vi "UPGRADE_Surge IFSM.vi"() -> ()   [LabVIEW 2019]
uses:
  <vilib>/Utility/NIReport.llb/Report Type.ctl
  <vilib>/Utility/NIReport.llb/NI_report.lvclass
  <vilib>/Utility/NIReport.llb/NI_ReportGenerationCore.lvlib
  <vilib>/Utility/NIReport.llb/Excel/NI_Excel.lvclass
panel:
  in  "Lot ID":string
  in  "Direction":string(combo)
  in  "Frequency (Hz)":i32
  in  "Temperature (+)":i32
  in  "Device ID":string
  in  "Technician":string
  in  "Request Number":i32
  out "STEP 8":bool
  out "STEP 7":bool
  out "STEP 6":bool
  out "STEP 5":bool
  in  "START Button":bool
  out "STEP 4":bool
  out "STEP 3":bool
  out "STEP 2":bool
  out "STEP 1":bool
  in  "FILE PATH":path
  # "DATA SUMMARY FOR SURGE IFSM"
  # "OPEN EXCEL FILE"
  # "RUN MACRO INTO EXCEL FILE"
  # "Create New Sheet named (Request Number_Surge_IFSM)"
  # "Create Table named (\"Last  Good Pass\")"
  # "Create New Sheet and Table named (\"Summary Table\")"
  # "Move All Tabs into a new Excel Workbook"
  # "SAVE EXCEL FILE"
  # "FINISH"
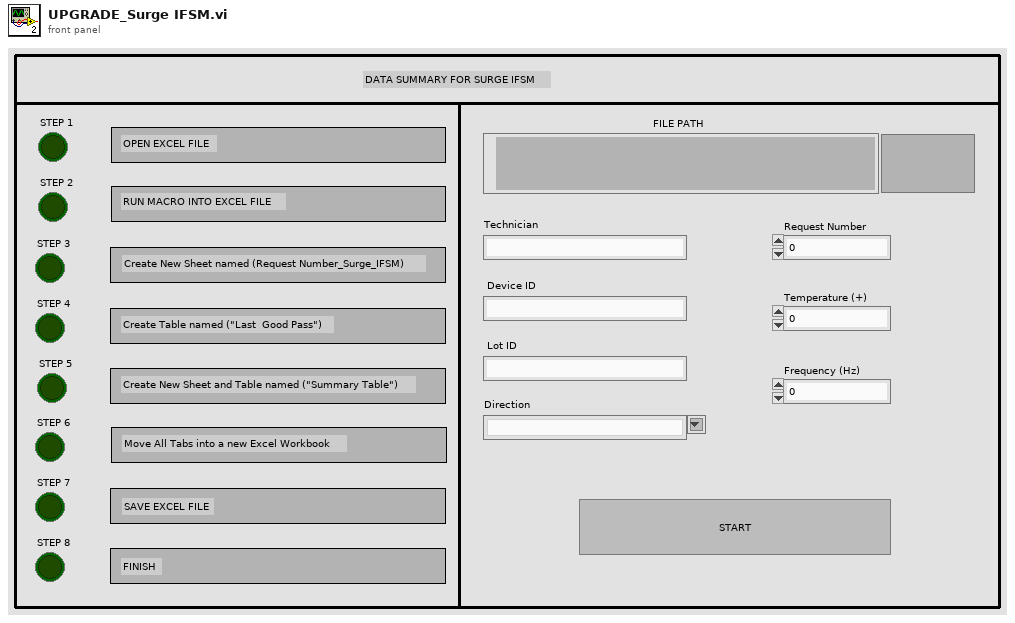
[diagram p1: front panel]
types:
  T1 = enum16{"maximized", "minimized", "normal", "no change"}
  T2 = typedef "NI_ReportGenerationCore.lvlib/Report Type.ctl" = enum16{"HTML", "Word", "Excel"}
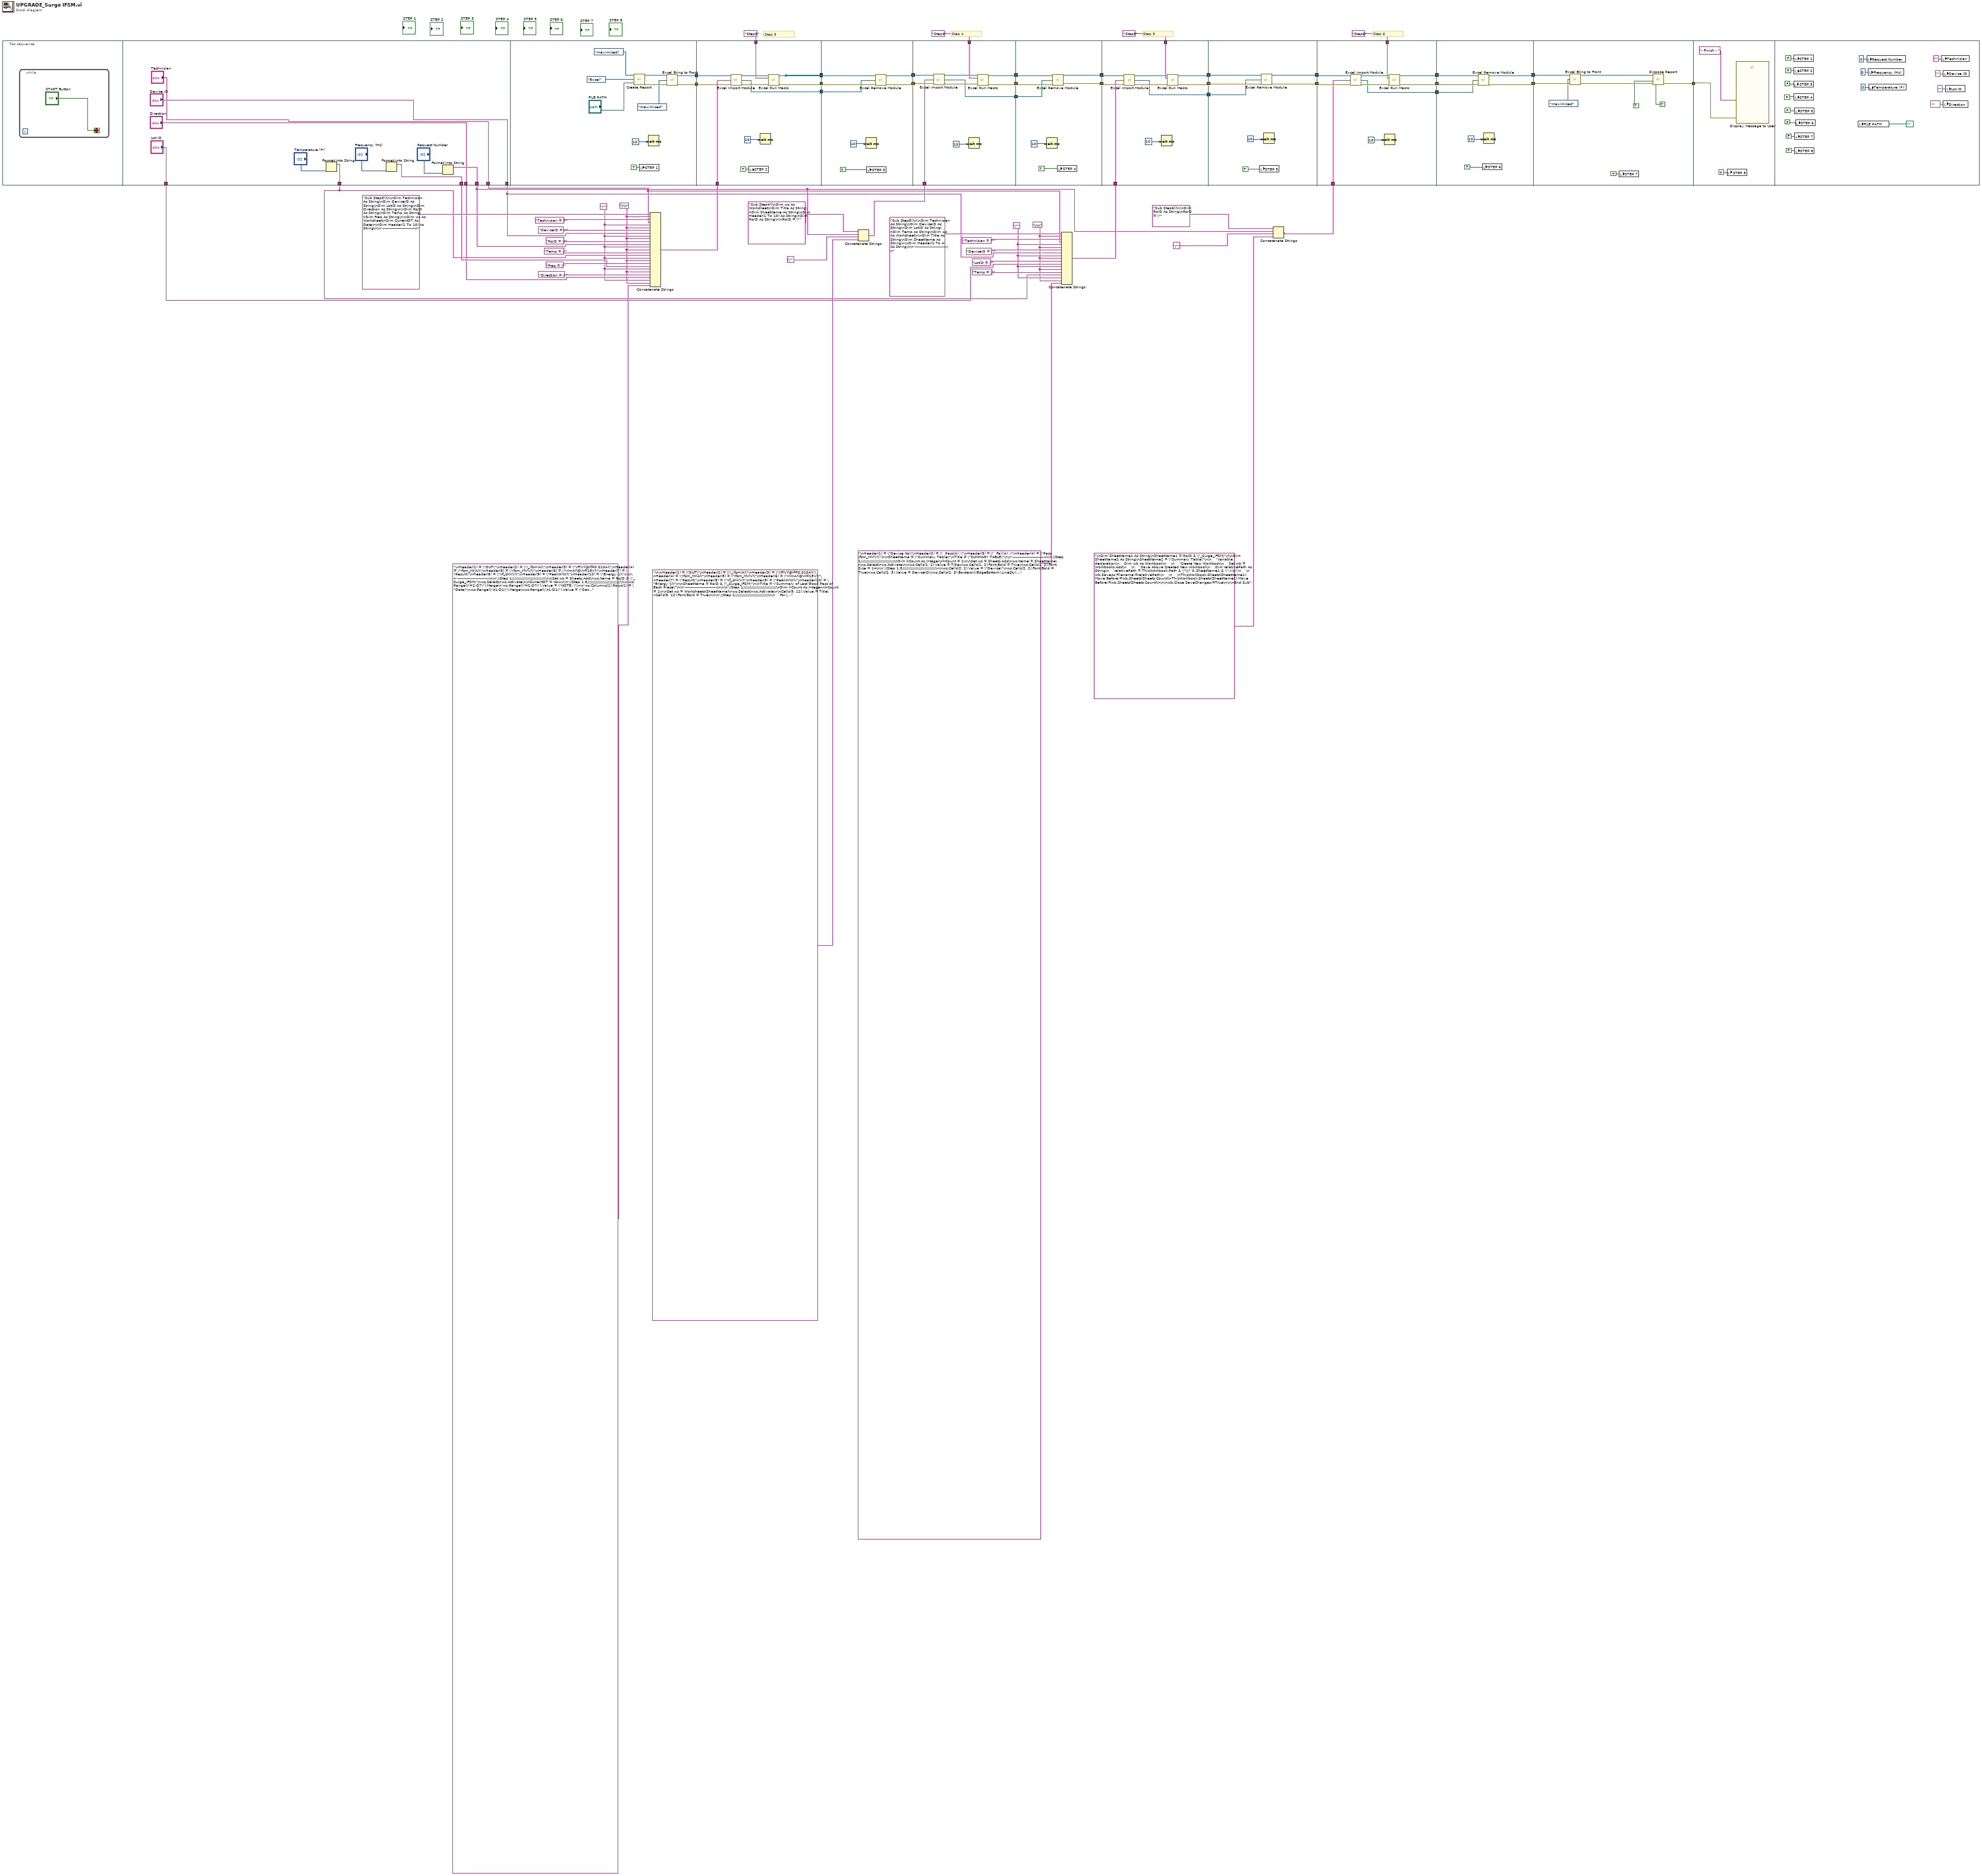
[diagram p0: block diagram]
diagram:
  w9 = "\r\n"
  w10 = "\"" ("string")
  w16 = "\r\n"
  w17 = "\"" ("string")
  # "Step 3"
  # "Step 6"
  # "Step 5"
  # "Step 4"
  n1 = flat-sequence {
    tunnel: [w73] -> w7
    tunnel: [w71] -> w6
    tunnel: [w69] -> w5
    tunnel: ["Direction"] -> w4
    tunnel: ["Device ID"] -> w3
    tunnel: ["Technician"] -> w2
    tunnel: ["Lot ID"] -> w1
    tunnel: [w77] -> w57
    tunnel: [w76] -> w56
    tunnel: [w93] -> w62
    tunnel: [w91] -> w61
    tunnel: "Step3" ("macro name") -> [w92]
    tunnel: [w91] -> w59
    tunnel: [w90] -> w58
    tunnel: w39 -> [w88]
    tunnel: w57 -> [w87]
    tunnel: w56 -> [w86]
    tunnel: w62 -> [w101]
    tunnel: [w99] -> w55
    tunnel: w61 -> [_]
    tunnel: [w100] -> w54
    tunnel: w59 -> [w102]
    tunnel: w58 -> [w98]
    tunnel: w55 -> [w109]
    tunnel: [w107] -> w53
    tunnel: w54 -> [w112]
    tunnel: [w110] -> w52
    tunnel: "Step4" ("macro name") -> [w106]
    tunnel: [w105] -> w40
    tunnel: w26 -> [w104]
    tunnel: w53 -> [w118]
    tunnel: w52 -> [w115]
    tunnel: [w117] -> w42
    tunnel: [w116] -> w41
    tunnel: w40 -> [w114]
    tunnel: [w124] -> w51
    tunnel: [w127] -> w50
    tunnel: w42 -> [w126]
    tunnel: w41 -> [w129]
    tunnel: "Step5" ("macro name") -> [w123]
    tunnel: [w122] -> w37
    tunnel: w36 -> [w121]
    tunnel: w51 -> [w135]
    tunnel: [w134] -> w47
    tunnel: w50 -> [w132]
    tunnel: [w133] -> w45
    tunnel: w37 -> [w131]
    tunnel: w47 -> [w146]
    tunnel: [w144] -> w46
    tunnel: w45 -> [w143]
    tunnel: [w141] -> w44
    tunnel: "Step6" ("macro name") -> [w140]
    tunnel: [w139] -> w34
    tunnel: w33 -> [w138]
    tunnel: w46 -> [w152]
    tunnel: [w151] -> w49
    tunnel: w44 -> [w150]
    tunnel: [w149] -> w48
    tunnel: w34 -> [w148]
    tunnel: w49 -> [w157]
    tunnel: w48 -> [w158]
    tunnel: [w161] -> w63
    tunnel: w63 -> [w163]
    frame #0 {
      n2 = while {
        stop <- "START Button" stop-if-true
      }
    }
    frame #1 {
      n3 = Format Into String("Temperature (+)") -> (resulting string=w69:string)  [unwired: 3 in, 1 out]
      n4 = Format Into String("Frequency (Hz)") -> (resulting string=w71:string)  [unwired: 3 in, 1 out]
      n5 = Format Into String("Request Number") -> (resulting string=w73:string)  [unwired: 3 in, 1 out]
    }
    frame #2 {
      n6 = call <vilib>:"Create Report.vi"("window state (normal)"=T1."maximized", "report type"=Report_Type."Excel", "template (empty)"="FILE PATH") -> ("report out"=w80:refnum<class "NI_report.lvclass">, "error out"=w81:errorcluster)  [unwired: 11 in]
      n7 = local write "STEP 1"(TRUE ("STEP 1")) -> ()
      n8 = Wait (ms)(milliseconds to wait=u32 10 ("millisecond timer value")) -> ()  [unwired: 1 out]
      n9 = call <vilib>:"Excel Bring to Front.vi"("report in"=w80, "window state (maximized)"=enum16{"maximized", "minimized", "normal"}."maximized", "error in (no error)"=w81) -> ("report out"=w77:refnum<class "NI_report.lvclass">, "error out"=w76:errorcluster)  [unwired: 11 in]
    }
    frame #3 {
      n10 = call <vilib>:"Excel Import Module.vi"("report in"=w87, "module code (\"\")"=w88, "error in (no error)"=w86) -> ("report out"=w95:refnum<class "NI_report.lvclass">, "module reference"=w90:refnum<k7>, "error out"=w94:errorcluster)  [unwired: 10 in]
      n11 = local write "STEP 2"(TRUE ("STEP 2")) -> ()
      n12 = Wait (ms)(milliseconds to wait=u32 10 ("millisecond timer value")) -> ()  [unwired: 1 out]
      n13 = call <vilib>:"Excel Run Macro.vi"("report in"=w95, "macro name"=w92, "error in (no error)"=w94) -> ("report out"=w91:refnum<class "NI_report.lvclass">, "error out"=w93:errorcluster)  [unwired: 10 in, 1 out]
    }
    frame #4 {
      n14 = Wait (ms)(milliseconds to wait=u32 10 ("millisecond timer value")) -> ()  [unwired: 1 out]
      n15 = local write "STEP 3"(TRUE) -> ()
      n16 = call <vilib>:"Excel Remove Module.vi"("report in"=w102, "module reference"=w98, "error in (no error)"=w101) -> ("report out"=w100:refnum<class "NI_report.lvclass">, "error out"=w99:errorcluster)  [unwired: 11 in]
    }
    frame #5 {
      n17 = call <vilib>:"Excel Import Module.vi"("report in"=w112, "module code (\"\")"=w104, "error in (no error)"=w109) -> ("report out"=w111:refnum<class "NI_report.lvclass">, "module reference"=w105:refnum<k7>, "error out"=w108:errorcluster)  [unwired: 10 in]
      n18 = Wait (ms)(milliseconds to wait=u32 10 ("millisecond timer value")) -> ()  [unwired: 1 out]
      n19 = call <vilib>:"Excel Run Macro.vi"("report in"=w111, "macro name"=w106, "error in (no error)"=w108) -> ("report out"=w110:refnum<class "NI_report.lvclass">, "error out"=w107:errorcluster)  [unwired: 10 in, 1 out]
    }
    frame #6 {
      n20 = Wait (ms)(milliseconds to wait=u32 10 ("millisecond timer value")) -> ()  [unwired: 1 out]
      n21 = call <vilib>:"Excel Remove Module.vi"("report in"=w115, "module reference"=w114, "error in (no error)"=w118) -> ("report out"=w116:refnum<class "NI_report.lvclass">, "error out"=w117:errorcluster)  [unwired: 11 in]
      n22 = local write "STEP 4"(TRUE) -> ()
    }
    frame #7 {
      n23 = call <vilib>:"Excel Import Module.vi"("report in"=w129, "module code (\"\")"=w121, "error in (no error)"=w126) -> ("report out"=w128:refnum<class "NI_report.lvclass">, "module reference"=w122:refnum<k7>, "error out"=w125:errorcluster)  [unwired: 10 in]
      n24 = Wait (ms)(milliseconds to wait=u32 10 ("millisecond timer value")) -> ()  [unwired: 1 out]
      n25 = call <vilib>:"Excel Run Macro.vi"("report in"=w128, "macro name"=w123, "error in (no error)"=w125) -> ("report out"=w127:refnum<class "NI_report.lvclass">, "error out"=w124:errorcluster)  [unwired: 10 in, 1 out]
    }
    frame #8 {
      n26 = local write "STEP 5"(TRUE) -> ()
      n27 = call <vilib>:"Excel Remove Module.vi"("report in"=w132, "module reference"=w131, "error in (no error)"=w135) -> ("report out"=w133:refnum<class "NI_report.lvclass">, "error out"=w134:errorcluster)  [unwired: 11 in]
      n28 = Wait (ms)(milliseconds to wait=u32 10 ("millisecond timer value")) -> ()  [unwired: 1 out]
    }
    frame #9 {
      n29 = call <vilib>:"Excel Import Module.vi"("report in"=w143, "module code (\"\")"=w138, "error in (no error)"=w146) -> ("report out"=w142:refnum<class "NI_report.lvclass">, "module reference"=w139:refnum<k7>, "error out"=w145:errorcluster)  [unwired: 10 in]
      n30 = Wait (ms)(milliseconds to wait=u32 10 ("millisecond timer value")) -> ()  [unwired: 1 out]
      n31 = call <vilib>:"Excel Run Macro.vi"("report in"=w142, "macro name"=w140, "error in (no error)"=w145) -> ("report out"=w141:refnum<class "NI_report.lvclass">, "error out"=w144:errorcluster)  [unwired: 10 in, 1 out]
    }
    frame #10 {
      n32 = call <vilib>:"Excel Remove Module.vi"("report in"=w150, "module reference"=w148, "error in (no error)"=w152) -> ("report out"=w149:refnum<class "NI_report.lvclass">, "error out"=w151:errorcluster)  [unwired: 11 in]
      n33 = local write "STEP 6"(TRUE) -> ()
      n34 = Wait (ms)(milliseconds to wait=u32 10 ("millisecond timer value")) -> ()  [unwired: 1 out]
    }
    frame #11 {
      n35 = call <vilib>:"Excel Bring to Front.vi"("report in"=w158, "window state (maximized)"=enum16{"maximized", "minimized", "normal"}."maximized", "error in (no error)"=w157) -> ("report out"=w155:refnum<class "NI_report.lvclass">, "error out"=w154:errorcluster)  [unwired: 11 in]
      n36 = local write "STEP 7"(TRUE ("STEP 3")) -> ()
      n37 = call-dynamic "Dispose Report.vi"("report in"=w155, "save changes? (F)"=TRUE, "error in (no error)"=w154, "close report? (T)"=TRUE) -> ("error out"=w161:errorcluster)  [unwired: 11 in]
    }
    frame #12 {
      n38 = local write "STEP 8"(TRUE ("STEP 4")) -> ()
      n39 = call "Display Message to User"("error in (no error)"=w163, "Message"="- Finish - ") -> ()  [unwired: 8 in, 2 out]
    }
    frame #13 {
      n40 = local write "STEP 3"(FALSE) -> ()
      n41 = local write "STEP 1"(FALSE ("STEP 1")) -> ()
      n42 = local write "STEP 2"(FALSE ("STEP 2")) -> ()
      n43 = local write "STEP 4"(FALSE) -> ()
      n44 = local write "STEP 5"(FALSE) -> ()
      n45 = local write "STEP 7"(FALSE ("STEP 3")) -> ()
      n46 = local write "STEP 8"(FALSE ("STEP 4")) -> ()
      n47 = local write "STEP 6"(FALSE) -> ()
      n48 = local write "FILE PATH"(path "" ("FILE PATH")) -> ()
      n49 = local write "Request Number"(0 ("Request Number")) -> ()
      n50 = local write "Frequency (Hz)"(0 ("Frequency (Hz)")) -> ()
      n51 = local write "Temperature (+)"(0 ("Temperature (+)")) -> ()
      n52 = local write "Technician"("" ("Technician")) -> ()
      n53 = local write "Device ID"("" ("Device ID")) -> ()
      n54 = local write "Direction"("" ("Direction")) -> ()
      n55 = local write "Lot ID"("" ("Lot ID")) -> ()
    }
  }
  n56 = Concatenate Strings("Sub Step3()\n\nDim Technician As String\nDim DeviceID As String\nDim LotID As String\nDim Direction As String\n\nDim RqID As String\nDim Temp As String\nDim Freq As String\n\nDim ws As Worksheet\nDim CurrentDT As Date\n\nDim Header(1 To 10) As String\n\n'---------------------------\n" ("string"), w16, "Technician = \"" ("string"), w2, w17, w16, "DeviceID = \"", w3, w17, w16, "RqID = \"", w7, w17, w16, "Temp = \"", w5, w17, w16, "Freq = \"", w6, w17, w16, "Direction = \"", w4, w17, w16, "\nHeader(1) = \"DUT\"\nHeader(2) = \"I_ifsm(A)\"\nHeader(3) = \"VF(V)(@If=0.010A)\"\nHeader(4) = \"Ifsm_MI(A)\"\nHeader(5) = \"Ifsm_MV(V)\"\nHeader(6) = \"Ir(mA)(@Vr=15V)\"\nHeader(7) = \"Result\"\nHeader(8) = \"Vf_chk(V)\"\nHeader(9) = \"PeakW(W)\"\nHeader(10) = \"Energy (J)\"\n\n\n'---------------------------\n\n'//Step 1////////////////////////////\n\nSet ws = Sheets.Add\nws.Name = RqID & \"_Surge_IFSM\"\nws.Select\nws.Activate\n\nCurrentDT = Now\n\n'//Step 1.5////////////////////////////\n\n'ws.Range(\"H2:O7\").Merge\n'ws.Range(\"H2:O7\").Value = \"NOTE: \"\n\n'ws.Columns(1).Rows(1) = \"Date\"\nws.Range(\"A1:D1\").Merge\nws.Range(\"A1:D1\").Value = \"Date\"\nws.Range(\"A1:D1\").HorizontalAlignment = xlRight\nws.Range(\"A1:D1\").Font.Bold = True\n\n'ws.Columns(1).Rows(2) = \"Time\"\nws.Range(\"A2:D2\").Merge\nws.Range(\"A2:D2\").Value = \"Time\"\nws.Range(\"A2:D2\").HorizontalAlignment = xlRight\nws.Range(\"A2:D2\").Font.Bold = True\n\n'ws.Columns(1).Rows(3) = \"Technician\"\nws.Range(\"A3:D3\").Merge\nws.Range(\"A3:D3\").Value = \"Technician\"\nws.Range(\"A3:D3\").HorizontalAlignment = xlRight\nws.Range(\"A3:D3\").Font.Bold = True\n\n'ws.Columns(1).Rows(4) = \"Device #\"\nws.Range(\"A4:D4\").Merge\nws.Range(\"A4:D4\").Value = \"Device #\"\nws.Range(\"A4:D4\").HorizontalAlignment = xlRight\nws.Range(\"A4:D4\").Font.Bold = True\n\n'ws.Columns(1).Rows(5) = \"Characterization #\"\nws.Range(\"A5:D5\").Merge\nws.Range(\"A5:D5\").Value = \"Characterization #\"\nws.Range(\"A5:D5\").HorizontalAlignment = xlRight\nws.Range(\"A5:D5\").Font.Bold = True\n\n'ws.Columns(1).Rows(6) = \"Temperature\"\nws.Range(\"A6:D6\").Merge\nws.Range(\"A6:D6\").Value = \"Temperature\"\nws.Range(\"A6:D6\").HorizontalAlignment = xlRight\nws.Range(\"A6:D6\").Font.Bold = True\n\n'ws.Columns(1).Rows(7) = \"Surge Type\"\nws.Range(\"A7:D7\").Merge\nws.Range(\"A7:D7\").Value = \"Surge Type\"\nws.Range(\"A7:D7\").HorizontalAlignment = xlRight\nws.Range(\"A7:D7\").Font.Bold = True\n\n'ws.Columns(1).Rows(8) = \"Surge Direction\"\nws.Range(\"A8:D8\").Merge\nws.Range(\"A8:D8\").Value = \"Surge Direction\"\nws.Range(\"A8:D8\").HorizontalAlignment = xlRight\nws.Range(\"A8:D8\").Font.Bold = True\n\n'ws.Columns(2).Rows(1) = Format(Now, \"mm/dd/yyyy\")\nws.Range(\"E1:G1\").Merge\nws.Range(\"E1:G1\").Value = Format(Now, \"mm/dd/yyyy\")\nws.Range(\"E1:G1\").HorizontalAlignment = xlLeft\n\n'ws.Columns(2).Rows(2) = Format(Now, \"HH:mm\")\nws.Range(\"E2:G2\").Merge\nws.Range(\"E2:G2\").Value = Format(Now, \"HH:mm\")\nws.Range(\"E2:G2\").HorizontalAlignment = xlLeft\n\n'ws.Columns(2).Rows(3) = Technician\nws.Range(\"E3:G3\").Merge\nws.Range(\"E3:G3\").Value = Technician\nws.Range(\"E3:G3\").HorizontalAlignment = xlLeft\n\n'ws.Columns(2).Rows(4) = DeviceID\nws.Range(\"E4:G4\").Merge\nws.Range(\"E4:G4\").Value = DeviceID\nws.Range(\"E4:G4\").HorizontalAlignment = xlLeft\n\n'ws.Columns(2).Rows(5) = RqID\nws.Range(\"E5:G5\").Merge\nws.Range(\"E5:G5\").Value = RqID\nws.Range(\"E5:G5\").HorizontalAlignment = xlLeft\n\n'ws.Columns(2).Rows(6) = \"+\" & Temp & \"C\"\nws.Range(\"E6:G6\").Merge\nws.Range(\"E6:G6\").Value = \"+\" & Temp & \"C\"\nws.Range(\"E6:G6\").HorizontalAlignment = xlLeft\n\n'ws.Columns(2).Rows(7) = Freq & \"Hz to Destruction (IFSM) \"\nws.Range(\"E7:G7\").Merge\nws.Range(\"E7:G7\").Value = Freq & \"Hz to Destruction (IFSM) \"\nws.Range(\"E7:G7\").HorizontalAlignment = xlLeft\n\n'ws.Columns(2).Rows(8) = Direction\nws.Range(\"E8:G8\").Merge\nws.Range(\"E8:G8\").Value = Direction\nws.Range(\"E8:G8\").HorizontalAlignment = xlLeft\n\n'ws.Range(\"A1:G8\").Columns.AutoFit\n'ws.Range(\"A1:G8\").HorizontalAlignment = xlRight\n\nws.Range(\"K2:R7\").Select\nws.Range(\"K2:R7\").Merge\nws.Range(\"K2:R7\").Value = \"NOTE: \"\nws.Range(\"K2:R7\").Borders.LineStyle = xlContinuous\nws.Range(\"K2:R7\").Borders.Weight = xlThick\n\nws.Range(\"K2:R7\").Font.Bold = True\nws.Range(\"K2:R7\").HorizontalAlignment = xlLeft\nws.Range(\"K2:R7\").VerticalAlignment = xlVAlignTop\n\n'//Step2////////////////////////////\n\n    For j = 1 To 10\n        Cells(9, j).Value = Header(j)\n    Next j\n\n\nRange(\"A9:J9\").Borders(xlEdgeBottom).Weight = xlThick\nRange(\"A9:J9\").Font.Bold = True\nRange(\"A9:J9\").Columns.AutoFit\n\n''//Step3 to 7////////////////////////////\n'\nDim CountFront As Integer\nDim SheetN As Integer\nDim msg As String\n\nSheetN = (Sheets.Count)\nCountFront = 0\nReDim Status(1 To SheetN) As String\n\n\n    '// Count how many available hastag\n    For j = 1 To SheetN\n\n             If Right(Sheets(j).Name, 1) = \"#\" Then\n             \n                                            If Len(Sheets(j).Name) = 2 Then\n                                            'MsgBox Left(Sheets(j).Name, 1)\n                                            Status(j) = Left(Sheets(j).Name, 1)\n                                            \n                                            ElseIf Len(Sheets(j).Name) = 3 Then\n                                            'MsgBox Left(Sheets(j).Name, 2)\n                                            Status(j) = Left(Sheets(j).Name, 2)\n                                            \n                                            ElseIf Len(Sheets(j).Name) = 4 Then\n                                            'MsgBox Left(Sheets(j).Name, 3)\n                                            Status(j) = Left(Sheets(j).Name, 3)\n                                            \n                                            End If\n'            CountFront = CountFront + 1\n            Else\n                Status(j) = 0\n            End If\n    Next j\n\n\n\n    '// Insert number(string) into array\n    Dim RowResultValue As Integer\n    Dim RowInputValue As Integer\n    Dim DUT As String\n    Dim StRange As String\n    Dim StLine As String\n\n\n    RowResultValue = 10\n    RowInputValue = 12\n    DUT = \" \"\n\n\n\n    For m = 1 To SheetN\n\n        If Status(m) = 0 Then\n\n        Else\n                    If Sheets(m).Columns(7).Rows(RowInputValue).Value <> \"FAIL\" Then\n\n                                Do While Sheets(m).Columns(7).Rows(RowInputValue).Value <> \"FAIL\"\n\n                                StRange = \"B\" & RowInputValue & \":J\" & RowInputValue\n\n                                ws.Columns(1).Rows(RowResultValue) = Status(m)\n                                Sheets(m).Range(StRange).Copy ws.Columns(2).Rows(RowResultValue)\n\n\n                                RowResultValue = RowResultValue + 1\n                                RowInputValue = RowInputValue + 1\n                                Loop\n                    End If\n\n\n\n                    If Sheets(m).Columns(7).Rows(RowInputValue).Value = \"FAIL\" Then\n\n                   \n\n\n                    StRange = \"B\" & RowInputValue & \":J\" & RowInputValue\n                    ws.Columns(1).Rows(RowResultValue) = Status(m)\n                    Sheets(m).Range(StRange).Copy ws.Columns(2).Rows(RowResultValue)\n\n                    StLine = \"A\" & RowResultValue & \":J\" & RowResultValue\n                    Range(StLine).Borders(xlEdgeBottom).Weight = xlThick\n\n                    RowResultValue = RowResultValue + 1\n                    RowInputValue = RowInputValue + 1\n\n                    Else\n\n                    MsgBox \" No Fail \"\n\n                    End If\n\n                    \n                    RowInputValue = 12\n        End If\n\n\n\n\n    Next m\n\n\n\n\nEnd Sub\n\n\n\n\n" ("string")) -> (w39:string)
  n57 = Concatenate Strings("Sub Step4()\nDim ws As Worksheet\nDim Title As String\nDim SheetName As String\nDim Header(1 To 10) As String\nDim RqID As String\n\nRqID = \"" ("string"), w7, "\"" ("string"), "\n\nHeader(1) = \"DUT\"\nHeader(2) = \"I_ifsm(A)\"\nHeader(3) = \"VF(V)(@If=0.010A)\"\nHeader(4) = \"Ifsm_MI(A)\"\nHeader(5) = \"Ifsm_MV(V)\"\nHeader(6) = \"Ir(mA)(@Vr=15V)\"\nHeader(7) = \"Result\"\nHeader(8) = \"Vf_chk(V)\"\nHeader(9) = \"PeakW(W)\"\nHeader(10) = \"Energy (J)\"\n\nSheetName = RqID & \"_Surge_IFSM\"\n\nTitle = \"Summary of Last Good Pass of Each Piece\"\n\n'---------------------------\n\n\n'//Step 1////////////////////////////\nDim hCount As Integer\nhCount = 1\n\nSet ws = Worksheets(SheetName)\nws.Select\nws.Activate\n\nCells(9, 12).Value = Title\nCells(9, 12).Font.Bold = True\n\n\n'//Step 2////////////////////////////\n\n    For j = 12 To 21\n        Cells(10, j).Value = Header(hCount)\n        hCount = hCount + 1\n    Next j\n\n\nRange(\"L10:U10\").Borders(xlEdgeBottom).Weight = xlThick\nRange(\"L10:U10\").Font.Bold = True\nRange(\"L10:U10\").Columns.AutoFit\n\n\n\n''//Step3 to 7////////////////////////////\n'\nDim CountFront As Integer\nDim SheetN As Integer\nDim msg As String\n\nSheetN = (Sheets.Count)\nCountFront = 0\nReDim Status(1 To SheetN) As String\n\n\n    '// Count how many available hastag\n    For j = 1 To SheetN\n\n             If Right(Sheets(j).Name, 1) = \"#\" Then\n             \n                                            If Len(Sheets(j).Name) = 2 Then\n                                            'MsgBox Left(Sheets(j).Name, 1)\n                                            Status(j) = Left(Sheets(j).Name, 1)\n                                            \n                                            ElseIf Len(Sheets(j).Name) = 3 Then\n                                            'MsgBox Left(Sheets(j).Name, 2)\n                                            Status(j) = Left(Sheets(j).Name, 2)\n                                            \n                                            ElseIf Len(Sheets(j).Name) = 4 Then\n                                            'MsgBox Left(Sheets(j).Name, 3)\n                                            Status(j) = Left(Sheets(j).Name, 3)\n                                            \n                                            End If\n'            CountFront = CountFront + 1\n            Else\n                Status(j) = 0\n            End If\n    Next j\n\n\n\n    '// Insert number(string) into array\n    Dim RowResultValue As Integer\n    Dim RowInputValue As Integer\n    Dim DUT As String\n    Dim StRange As String\n    Dim StLine As String\n\n\n    RowResultValue = 11\n    RowInputValue = 12\n    DUT = \" \"\n\n\n\n    For m = 1 To SheetN\n\n        If Status(m) = 0 Then\n\n        Else\n                    If Sheets(m).Columns(7).Rows(RowInputValue).Value <> \"FAIL\" Then\n\n                                Do While Sheets(m).Columns(7).Rows(RowInputValue).Value <> \"FAIL\"\n                                RowInputValue = RowInputValue + 1\n                                Loop\n                    End If\n\n\n\n                    If Sheets(m).Columns(7).Rows(RowInputValue).Value = \"FAIL\" Then\n\n                \n\n                    StRange = \"B\" & (RowInputValue - 1) & \":J\" & (RowInputValue - 1)\n                    ws.Columns(12).Rows(RowResultValue) = Status(m)\n                    Sheets(m).Range(StRange).Copy ws.Columns(13).Rows(RowResultValue)\n\n                    RowResultValue = RowResultValue + 1\n                    RowInputValue = RowInputValue + 1\n\n                    Else\n\n                    MsgBox \" No Fail \"\n\n                    End If\n\n                    \n                    RowInputValue = 12\n        End If\n\n\n\n\n    Next m\n\n\n\nEnd Sub\n\n\n\n\n" ("string")) -> (w26:string)
  n58 = Concatenate Strings("Sub Step5()\n\nDim Technician As String\nDim DeviceID As String\nDim LotID As String\nDim Temp As String\nDim ws As Worksheet\n\nDim Title As String\nDim SheetName As String\n\nDim Header(1 To 4) As String\n\n'---------------------------\n" ("string"), w9, "Technician = \"" ("string"), w2, w10, w9, "DeviceID = \"", w3, w10, w9, "LotID = \"", w1, w10, w9, "Temp = \"", w5, w10, w9, "\nHeader(1) = \"Device No\"\nHeader(2) = \"  Pass(A)  \"\nHeader(3) = \"  Fail(A)  \"\nHeader(4) = \"Pass Ifsm_MV(V)\"\n\nSheetName = \"Summary Table\"\nTitle = \"SUMMARY TABLE\"\n\n'---------------------------\n\n'//Step 1////////////////////////////\nDim hCount As Integer\nhCount = 1\n\nSet ws = Sheets.Add\nws.Name = SheetName\nws.Select\nws.Activate\n\nws.Cells(1, 2).Value = Title\nws.Cells(1, 2).Font.Bold = True\nws.Cells(1, 2).Font.Size = 14\n\n'//Step 1.5////////////////////////////\n\nws.Cells(2, 2).Value = \"Device\"\nws.Cells(2, 2).Font.Bold = True\nws.Cells(2, 3).Value = DeviceID\nws.Cells(2, 3).Borders(xlEdgeBottom).LineStyle = xlContinuous\nws.Cells(2, 4).Borders(xlEdgeBottom).LineStyle = xlContinuous\n\nws.Cells(3, 2).Value = \"Technician\"\nws.Cells(3, 2).Font.Bold = True\nws.Cells(3, 3).Value = Technician\nws.Cells(3, 3).Borders(xlEdgeBottom).LineStyle = xlContinuous\nws.Cells(3, 4).Borders(xlEdgeBottom).LineStyle = xlContinuous\n\nws.Cells(4, 2).Value = \"LOT #\"\nws.Cells(4, 2).Font.Bold = True\nws.Cells(4, 3).Value = LotID\nws.Cells(4, 3).Borders(xlEdgeBottom).LineStyle = xlContinuous\nws.Cells(4, 4).Borders(xlEdgeBottom).LineStyle = xlContinuous\n\nws.Cells(2, 6).Value = \"Sample Type\"\nws.Cells(2, 6).Font.Bold = True\nws.Cells(2, 7).Value = \"Diode_N\"\nws.Cells(2, 7).Borders(xlEdgeBottom).LineStyle = xlContinuous\n\n\nws.Cells(3, 6).Value = \"Wave\"\nws.Cells(3, 6).Font.Bold = True\nws.Cells(3, 7).Value = \"Sine\"\nws.Cells(3, 7).Borders(xlEdgeBottom).LineStyle = xlContinuous\n\n\nws.Cells(2, 9).Value = \"Temperature\"\nws.Cells(2, 9).Font.Bold = True\nws.Cells(2, 10).Value = Temp & \"C\"\nws.Cells(2, 10).Borders(xlEdgeBottom).LineStyle = xlContinuous\n\n\nws.Cells(3, 9).Value = \"Width\"\nws.Cells(3, 9).Font.Bold = True\nws.Cells(3, 10).Value = \"8.3ms\"\nws.Cells(3, 10).Borders(xlEdgeBottom).LineStyle = xlContinuous\n\nws.Range(\"B2:J4\").Columns.AutoFit\n\n'//Step 2////////////////////////////\n\n    For j = 2 To 5\n        Cells(6, j).Value = Header(hCount)\n        hCount = hCount + 1\n    Next j\n\n\nRange(\"B6:E6\").Borders(xlEdgeBottom).Weight = xlThick\nRange(\"B6:E6\").Borders.LineStyle = xlContinuous\nRange(\"B6:E6\").Font.Bold = True\nRange(\"B6:E6\").Columns.AutoFit\nRange(\"B6:E6\").Interior.ColorIndex = 6 'Yellow\n\n\n'//Step3 to 7////////////////////////////\n'\nDim CountFront As Integer\nDim SheetN As Integer\nDim msg As String\n\nSheetN = (Sheets.Count)\nCountFront = 0\nReDim Status(1 To SheetN) As String\n\n\n    '// Count how many available hastag\n    For j = 1 To SheetN\n\n             If Right(Sheets(j).Name, 1) = \"#\" Then\n\n                                            If Len(Sheets(j).Name) = 2 Then\n                                            'MsgBox Left(Sheets(j).Name, 1)\n                                            Status(j) = Left(Sheets(j).Name, 1)\n\n                                            ElseIf Len(Sheets(j).Name) = 3 Then\n                                            'MsgBox Left(Sheets(j).Name, 2)\n                                            Status(j) = Left(Sheets(j).Name, 2)\n\n                                            ElseIf Len(Sheets(j).Name) = 4 Then\n                                            'MsgBox Left(Sheets(j).Name, 3)\n                                            Status(j) = Left(Sheets(j).Name, 3)\n\n                                            End If\n'            CountFront = CountFront + 1\n            Else\n                Status(j) = 0\n            End If\n    Next j\n\n\n\n    '// Insert number(string) into array\n    Dim RowResultValue As Integer\n    Dim RowInputValue As Integer\n    Dim DUT As String\n    Dim StRange As String\n    Dim StLine As String\n\n    Dim StPass As String\n    Dim StFail As String\n    Dim StIfsmPass As String\n    Dim St4Border As String\n\n    RowResultValue = 7\n    RowInputValue = 12\n    DUT = \" \"\n\n\n\n    For m = 1 To SheetN\n\n        If Status(m) = 0 Then\n\n        Else\n                    If Sheets(m).Columns(7).Rows(RowInputValue).Value <> \"FAIL\" Then\n\n                                Do While Sheets(m).Columns(7).Rows(RowInputValue).Value <> \"FAIL\"\n                                RowInputValue = RowInputValue + 1\n                                Loop\n                    End If\n\n\n\n                    If Sheets(m).Columns(7).Rows(RowInputValue).Value = \"FAIL\" Then\n\n                   \n\n                    StPass = \"C\" & (RowInputValue - 1)\n                    StFail = \"C\" & (RowInputValue)\n                    StIfsmPass = \"F\" & (RowInputValue - 1)\n                    St4Border = \"B\" & (RowResultValue) & \":E\" & (RowResultValue)\n\n                    ws.Columns(2).Rows(RowResultValue) = Status(m) 'DUT\n                    ws.Columns(3).Rows(RowResultValue) = Sheets(m).Range(StPass) 'PASS\n                    ws.Columns(4).Rows(RowResultValue) = Sheets(m).Range(StFail) 'FAIL\n                    ws.Columns(5).Rows(RowResultValue) = Sheets(m).Range(StIfsmPass) 'Pass Ifsm_MV(V)\n                    ws.Range(St4Border).Borders.LineStyle = xlContinuous\n\n                    RowResultValue = RowResultValue + 1\n                    RowInputValue = RowInputValue + 1\n\n                    Else\n\n                    MsgBox \" No Fail \"\n\n                    End If\n\n\n                    RowInputValue = 12\n        End If\n\n\n\n\n    Next m\n\n\n\nEnd Sub\n\n" ("string")) -> (w36:string)
  n59 = Concatenate Strings("Sub Step6()\n\nDim RqID As String\nRqID = \"" ("string"), w7, "\"" ("string"), "\nDim SheetName1 As String\nSheetName1 = RqID & \"_Surge_IFSM\"\n\nDim SheetName2 As String\nSheetName2 = \"Summary Table\"\n\n    'Variable declaration\n    Dim wb As Workbook\n    \n    'Create New Workbook\n    Set wb = Workbooks.Add\n    \n    'Save Above Created New Workbook\n    Dim relativePath As String\n    relativePath = ThisWorkbook.Path & \"\\\" & SheetName1 & \".xls\"\n    \n    wb.SaveAs Filename:=relativePath\n    \n    \nThisWorkbook.Sheets(SheetName1).Move Before:=wb.Sheets(Sheets.Count)\nThisWorkbook.Sheets(SheetName2).Move Before:=wb.Sheets(Sheets.Count)\n\n\nwb.Close SaveChanges:=True\n\n\nEnd Sub" ("string")) -> (w33:string)
